vi "DefendAreaTactic.vi"(6 "Number of Defenders\nWithout Duelist":i32, 7 "First call?":bool, 8 "error in (no error)":errorcluster, 9 "Robot":refnum<class "Robot.lvclass">, 10 "Game in":refnum<class "Game.lvclass">, 11 "DefendAreaTactic in":refnum<class "DefendAreaTactic.lvclass">) -> (0 "error out":errorcluster, 2 "Robot out":refnum<class "Robot.lvclass">, 3 "DefendAreaTactic out":refnum<class "DefendAreaTactic.lvclass">)   [LabVIEW 2024, in "DefendAreaTactic.lvclass"]
uses:
  DefendAreaTactic.lvclass
  C:/Users/moise/Documents/GitHub/SSL_AI/Tactic_class/Tactic.lvclass
  Robot_class/Robot.lvclass
  C:/Users/moise/Documents/GitHub/SSL_AI/Object_class/Object.lvclass
  Game_class/Game.lvclass
  Robot_class/tactics.ctl
  DefendAreaTacticStates.ctl
  Robot_class/robotKickToStates.ctl
  Tactic_class/Tactic.lvclass/Tactic.ctl
  WallPositions.ctl
  Robot_class/Robot.lvclass/Robot.ctl
  Object_class/Object.lvclass/Object.ctl
  Game_class/Game.lvclass/Game.ctl
  Team_class/Team.lvclass/Team.ctl
  Ball_class/Ball.lvclass/Ball.ctl
  Field_class/Field.lvclass/Field.ctl
  Parameters_class/Parameters.lvclass/Parameters.ctl
  Skillbook_class/Skillbook.lvclass/Skillbook.ctl
  DefendAreaTactic.lvclass/DefendAreaTactic.ctl
  <vilib>/Analysis/_algsub.llb/Real Vector Norm.vi
  Game_class/Read DefensiveTeam.vi
  Game_class/Read BallRef.vi
  Game_class/Read FieldRef.vi
  Game_class/Read NewParameters.vi
  Field_class/Read ourGoalPosition.vi
  Ball_class/Read v_x.vi
  Ball_class/Read v_y.vi
  Object_class/Read x.vi
  Object_class/Read y.vi
  Object_class/Read position(x,y).vi
  Ball_class/Read velocityNorm.vi
  Team_class/Read RobotRef.vi
  Robot_class/Read id.vi
  Robot_class/Write dest_x.vi
  Robot_class/Write dest_y.vi
  Robot_class/Write dest_orientation.vi
  Game_class/Read OffensiveTeam.vi
  Game_class/Read EnemyRef.vi
  Game_class/Read Parameters.lvclass.vi
  Game_class/Read Utilities.lvclass.vi
  Parameters_class/Read AttakingOurselves.vi
  Skillbook_class/Read HaltSkill.vi
  Tactic_class/Read Skillbook.vi
  Write States.vi
  Robot_class/Write tactic.vi
  Robot_class/Write keepDest.vi
  Robot_class/Write robotKickState.vi
  Ball_class/Ball.lvclass
  Ally_class/Ally.lvclass
  C:/Users/moise/Documents/GitHub/SSL_AI/Team_class/Team.lvclass
  Enemy_class/Enemy.lvclass
  Skillbook_class/Skillbook.lvclass
  Field_class/Field.lvclass
  Parameters_class/Parameters.lvclass
  Utilities_class/Utilities.lvclass
  HaltSkill_class/HaltSkill.lvclass
  DefendGoalTactic_class/DefendGoalTactic.lvclass
  <vilib>/Analysis/NI_AALPro.lvlib
  <vilib>/Analysis/coordinate.llb/2D Cartesian Coordinate Rotation (Scalar).vi
  Team_class/Team.lvclass
  <vilib>/Analysis/NI_AALBLAS.lvlib
panel:
  out "x .or. y?":bool
  out "Dist":dbl
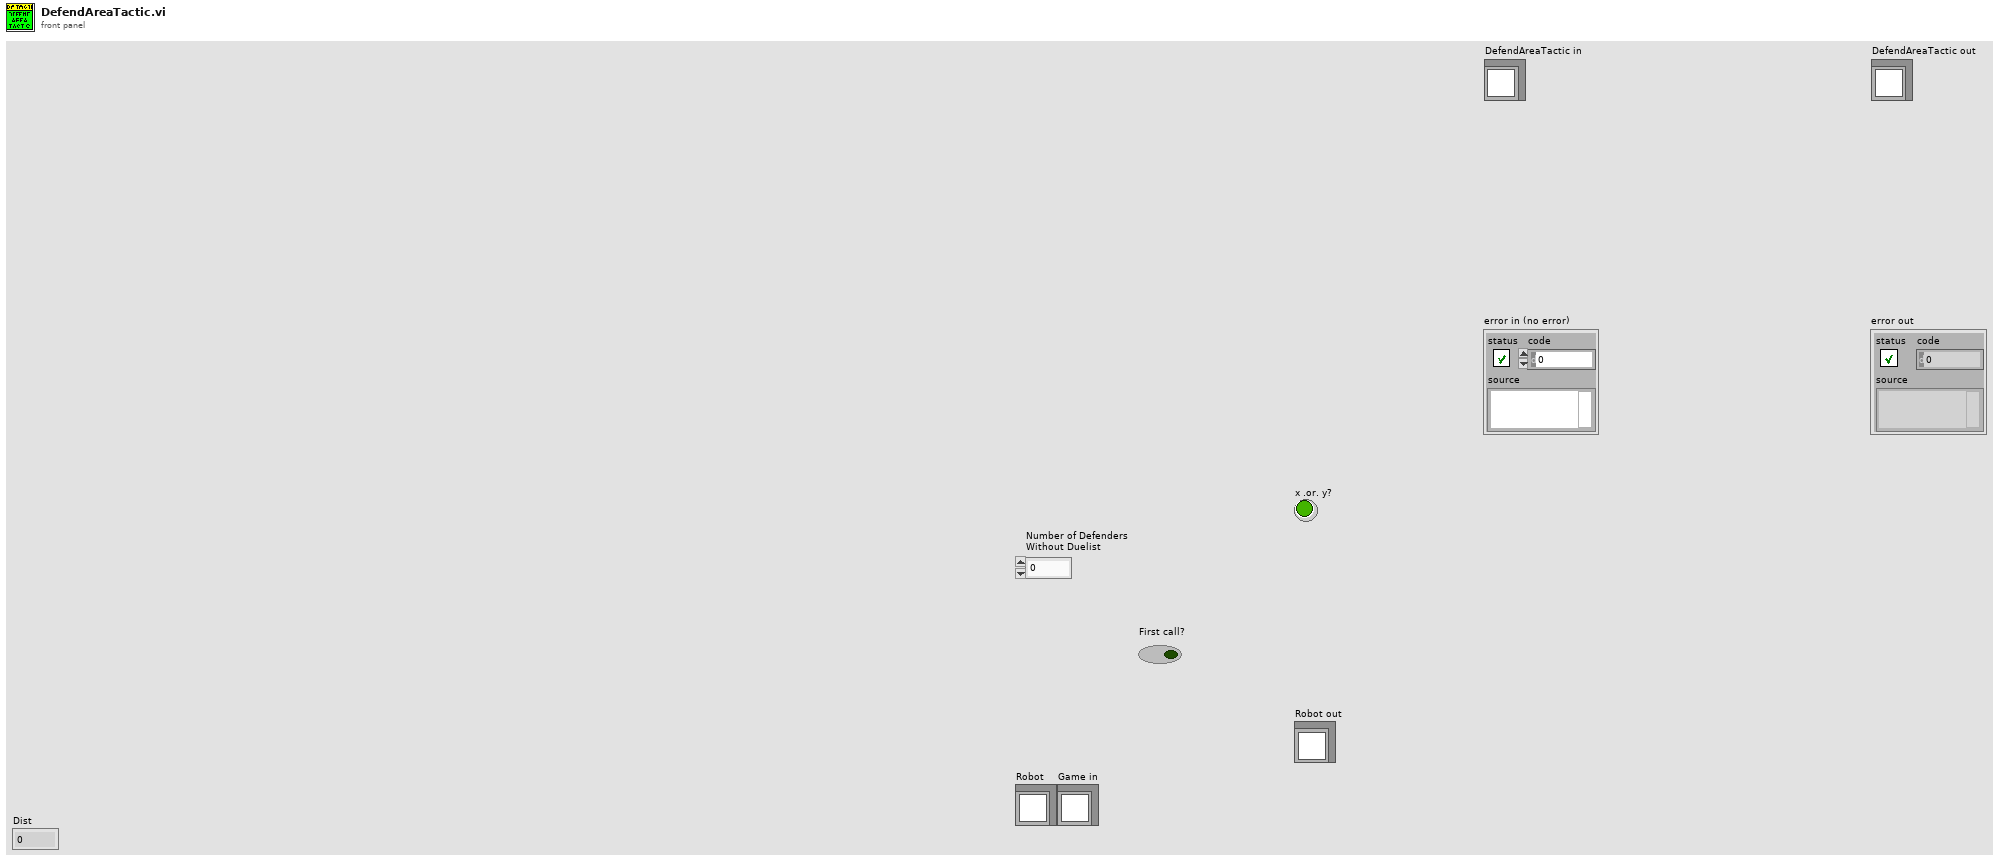
[diagram p1: front panel]
types:
  T1 = typedef "robotKickToStates.ctl" = enum16{"shootFromDirect", "avoidCollideBall", "goToBackBall", "none", "walk", "turn", "turnAntiClockWise", "turnClockwise", "oldKickToShoot", "oldKickToGoToBackBall", "shoot"}
  T2 = typedef "DefendAreaTactic.lvclass/DefendAreaTacticStates.ctl" = enum16{"BlockShot", "BlockPossibleShot", "CoverOneTouchShot", "BallInKeeperArea", "Exit"}
  T3 = typedef "tactics.ctl" = enum16{"GoToBallPlacementPosition", "PlaceBall", "GoToBallPlacement", "5Robots", "BallPlacementEnemy", "ReceivePassInFuturePoint", "Roller", "PrepareRollToPassRollerGoTo", "PrepareRollToPassReceiverGoTo", "WaitRoll", "PositionToRoll", "PenaltyAttacker", "PassObserver", "PenaltyDefense", "TableReceiverTactic", "Test", "DefendGoal", "Marker", "FollowAttacker", "DefendArea", "Shoot", "AttackerAimGoal", "AttackerBallOutOfField", "AttackerBlock", "AttackerStop", "Duelist", "Halt", "ZigZag", "GoTo", "Timeout", "KickToBestRobot", "KickToPassReceiver", "PositionToReceivePass", "WaitPass", "GoToTarget"}
  T4 = typedef "WallPositions.ctl" = enum16{"LeftWall", "LeftCorner", "FrontWall", "RightCorner", "RightWall"}
  T5 = typedef "NewParameters.ctl" = cluster{"PenaltyDistance":dbl, "DistanceAttackerToBackBall":dbl, "Division":enum16{"Div B", "Div A"}, "DistanceToAvoidyEnemyRobot":dbl, "BallPlacementDistance":dbl, "DisatanceBehindBallToStealBall":dbl, "MaxDistanceToPositionKickoff":dbl, "BlockEnemyTarget":bool, "MaxStopVAng":dbl, "DistanceMarkerToEnemy":dbl, "IgnoreDribblerContact":bool, "DistanceToBeginEnemyPosession":dbl, "GoToBallWhenEnemyNotMoving":bool, "EnemyDistanceToReduceVelocity":dbl, "TurnOnEnemyDistanceToReduceVelocity":bool, "EnemyDistanceToShootOutBall":dbl, "DefenseKickBall":bool, "MoreKickToGoal? (0-0.3)":dbl, "ChipKickInEnemyField":bool, "ShootOutRobotId":dbl, "FieldLenghtDenominatorInShootOut":dbl, "AdjustPositionInBallPlacement":bool, "PowerGodPass":dbl, "VelocityAbortEnemyPos":dbl, "MaxDistToBeginPass":dbl, "MinDistToBeginPass":dbl, "VelocityInDirects":dbl, "BadDribblerIDs":i32[], "NewKickToDistanceAroundBall":dbl, "PowerAvoidColisionMarker":dbl, "DistanceToAvoidColisionMarker":dbl, "AvoidBallKick":dbl, "DistanceTryKick":dbl, "SuicideKickDIstance":dbl, "AdjustFirstKickDistance":dbl, "AvoidAimLessKick":dbl, "DistanceToAvoidyEnemyShootRobot ":dbl, "NumberOfMarkers":dbl, "PotField":bool, "PIDLateral":bool, "MinDistanceFirstKickX":dbl, "MinDistanceFirstKickY":dbl, "FractionOfDistToTouchGround\nAfterChipKick":dbl, "FractionOfKickxWhen\nComposedWithKickz":dbl, "Style":T6, "MoveInTurnState":bool, "DistFromEnemyToConsider\nMoveInTurnState":dbl, "CascadePID":bool, "TurnAroundParameters":cluster{"Radius":dbl, "Multiplier":dbl, "ChordAngle":dbl}, "SafeDriveVel":dbl, "DistanceToGoToBackBall":dbl, "minDistanceToNotFinish\nEnemyPossession":dbl, "OneTouchShot":cluster{"angleFactor":dbl, "maxAngle":dbl, "Attack":bool, "Defense":bool}, "OpenAngleToGoal":cluster{"minAngle":dbl, "maxAngle":dbl, "minEvaluation":dbl}, "ShotInterception":cluster{"shotSpeed":dbl, "minEnemySpeed":dbl, "maxEnemySpeed":dbl, "minEvaluation":dbl}, "AllyTeamArray":T7[], "maxDefendersNumber":i32, "Zone":cluster{"GuardPositionArray":dbl[][], "ZoneMidField":dbl[], "CenterForwardWidth":dbl}, "MinEvaluationToShoot":dbl, "PassInterception":cluster{"maxPassSpeed":dbl, "minPassSpeed":dbl, "minEnemySpeed":dbl, "chipPassDistance":dbl, "chipPassEvaluation":dbl, "minEvaluation":dbl, "maxEnemySpeed":dbl}, "PassDistance":cluster{"maxDistance":dbl, "minDistance":dbl}, "receiverSpeed":dbl, "maxBallSpeed":dbl, "slackTime":dbl, "Turning radius":dbl, "Turning v_ang":dbl, "AlignError":cluster{"Distance":dbl, "Orientation":dbl, "V_norm(m/s)":dbl, "V_ang (rad/s)":dbl}, "RobotRadius":dbl, "KickerDistance":dbl, "keeper angle  to cover goalpost":dbl, "a_slide":dbl, "a_roll":dbl, "k_switch":dbl}
  T6 = typedef "Style.ctl" = enum16{"Insanity", "Offensive", "Defensive"}
  T7 = typedef "AllyTeam.ctl" = enum16{"Keeper", "Defender", "Attacker"}
  T8 = typedef "DefendGoalTactic.lvclass/DefendGoalTacticStates.ctl" = enum16{"BlockShot", "BlockPossibleShot", "CoverOneTouchShot", "Kick", "GuardGoal", "Exit"}
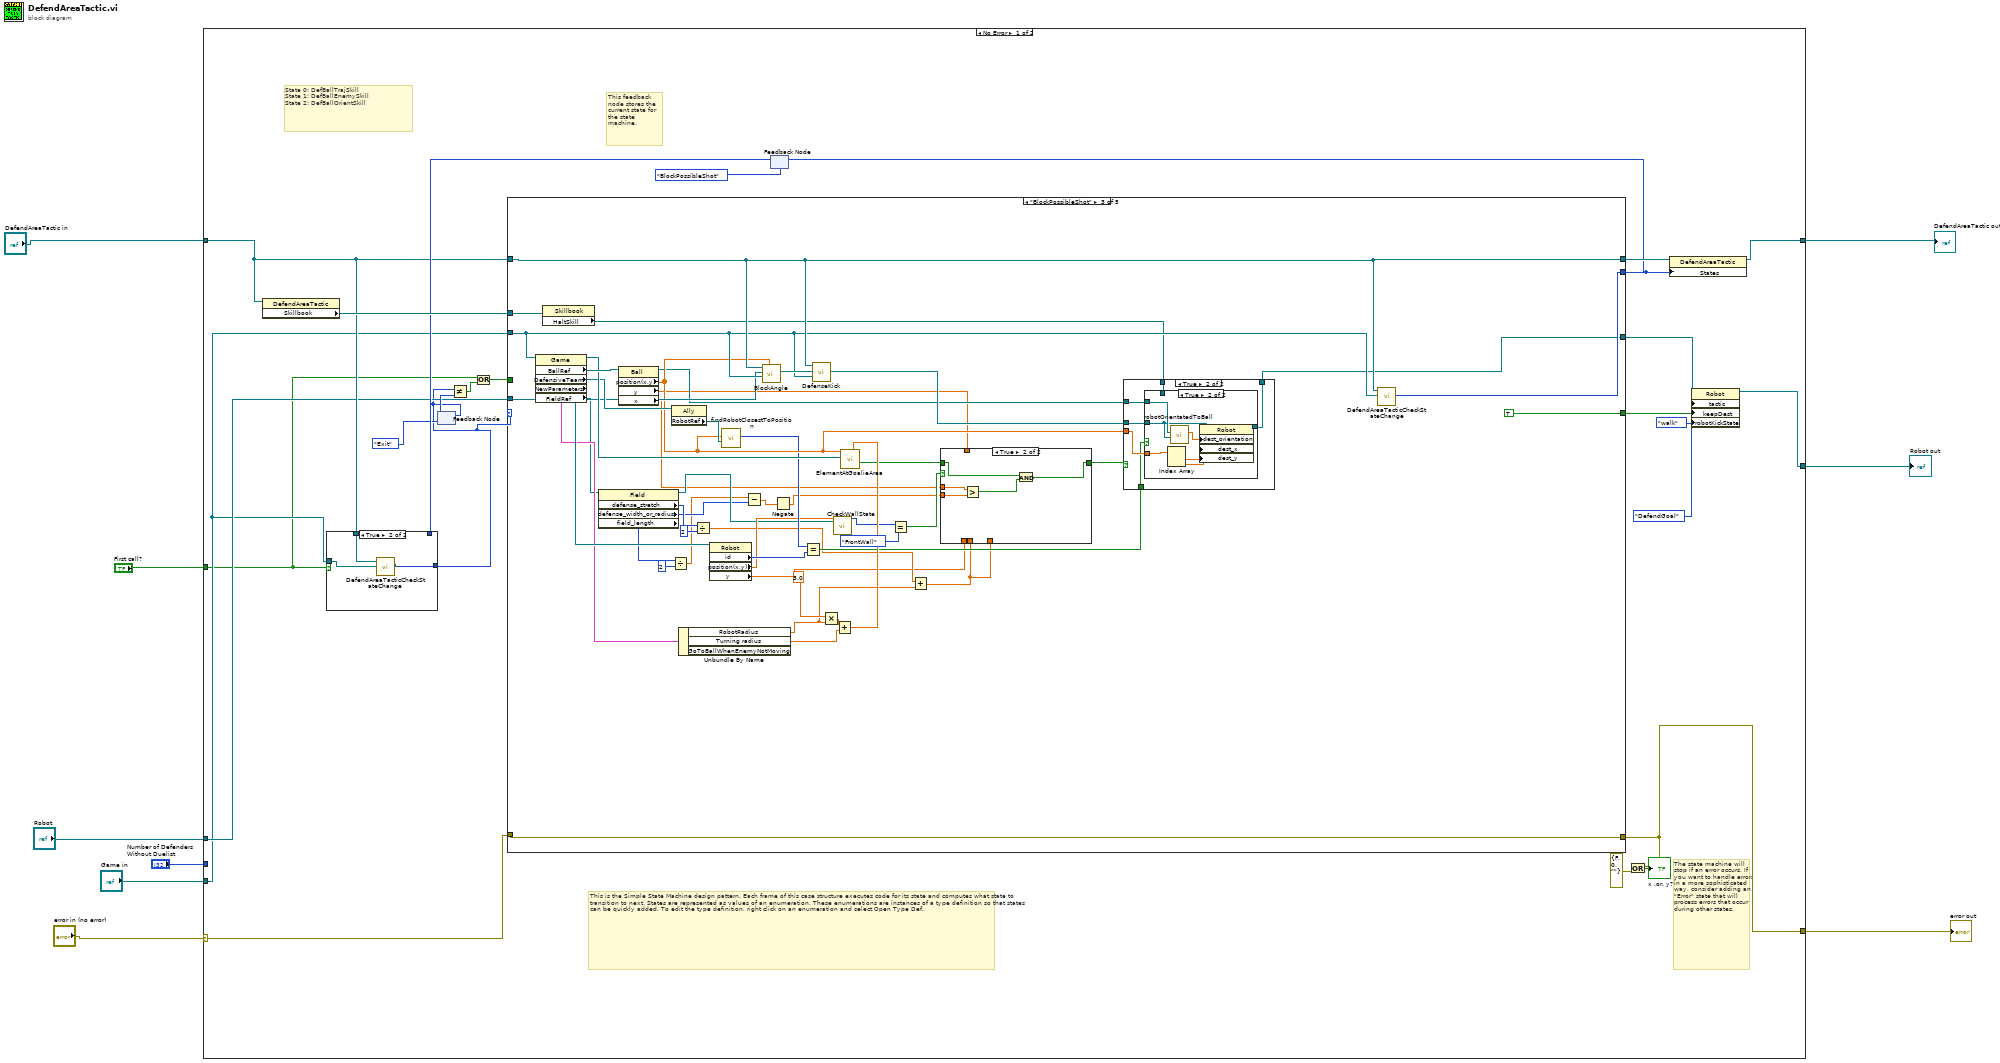
[diagram p0: block diagram]
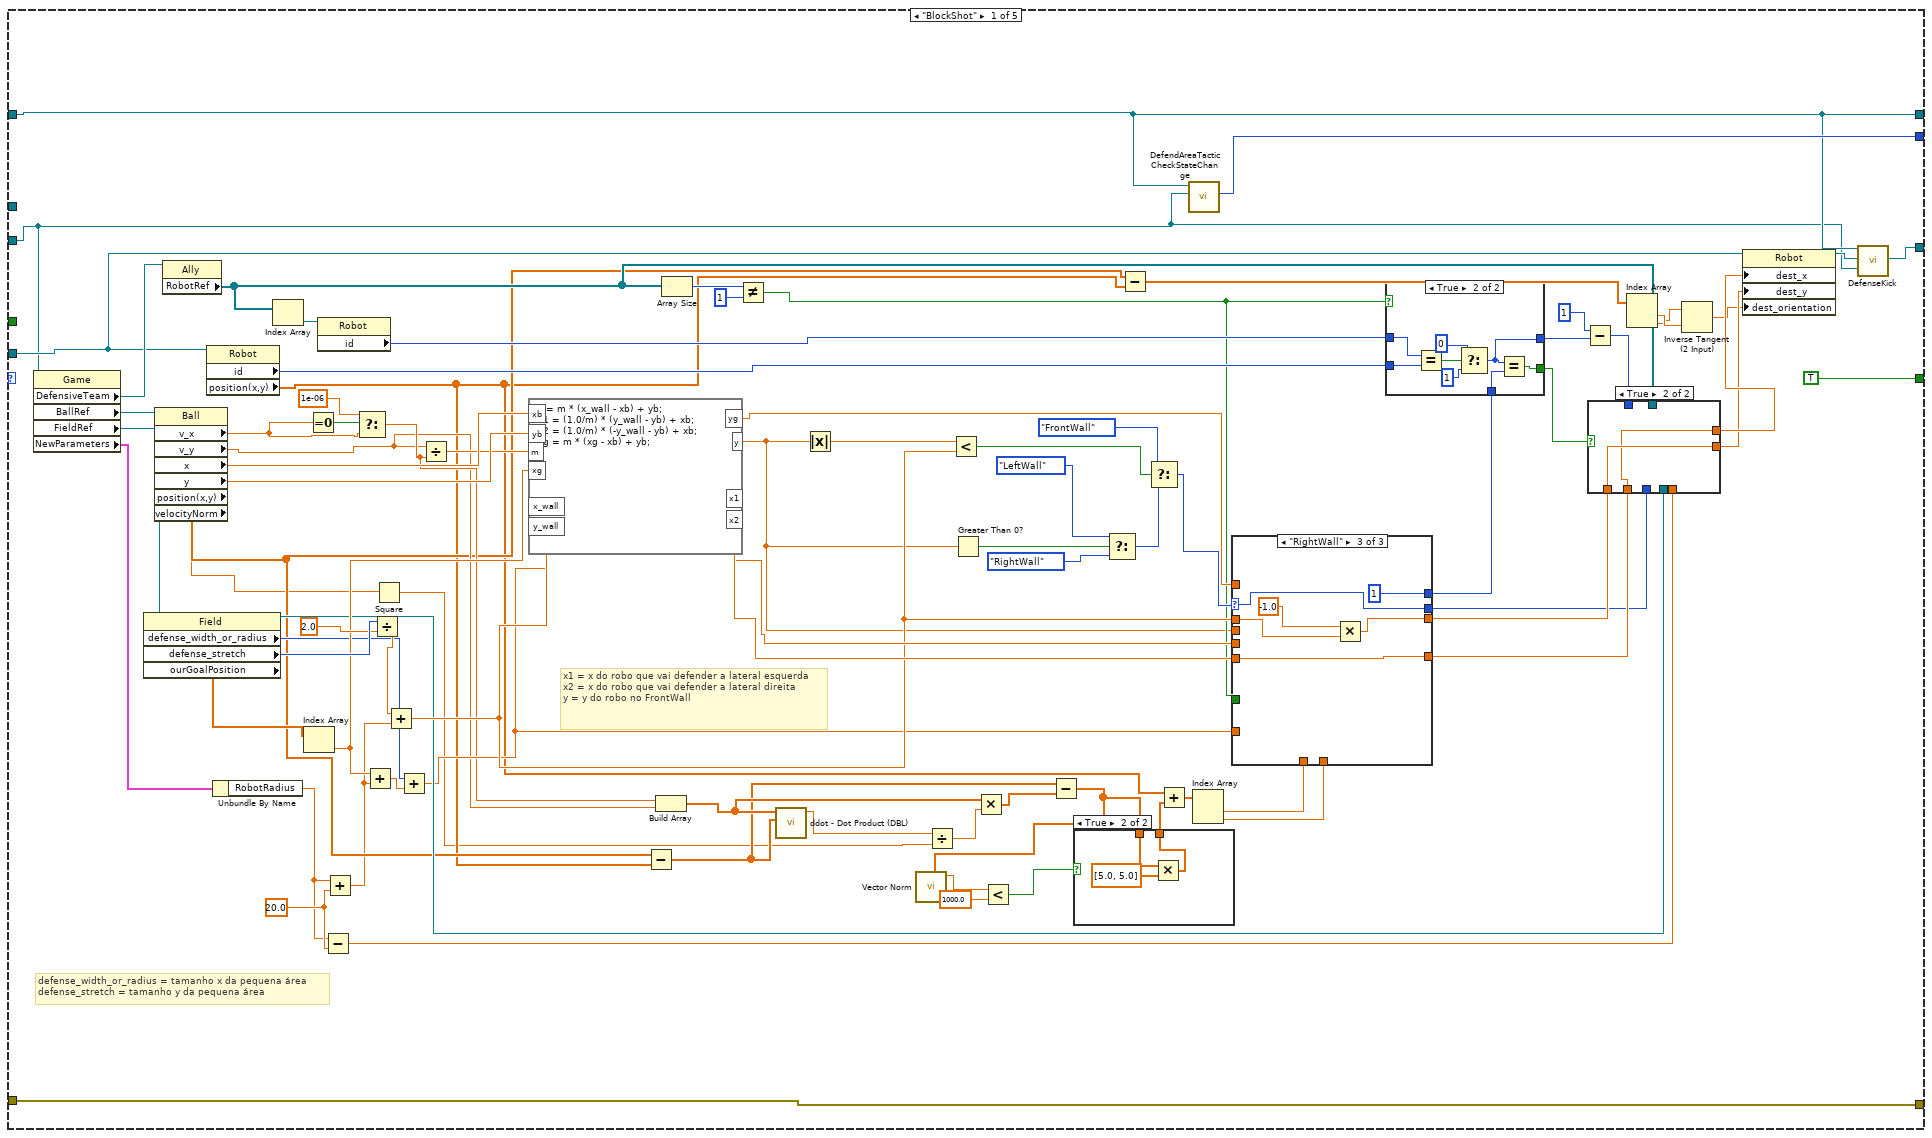
[diagram p3: hidden frame]
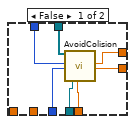
[diagram p5: hidden frame]
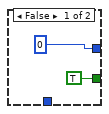
[diagram p6: hidden frame]
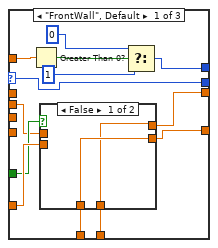
[diagram p7: hidden frame]
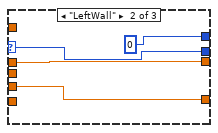
[diagram p9: hidden frame]
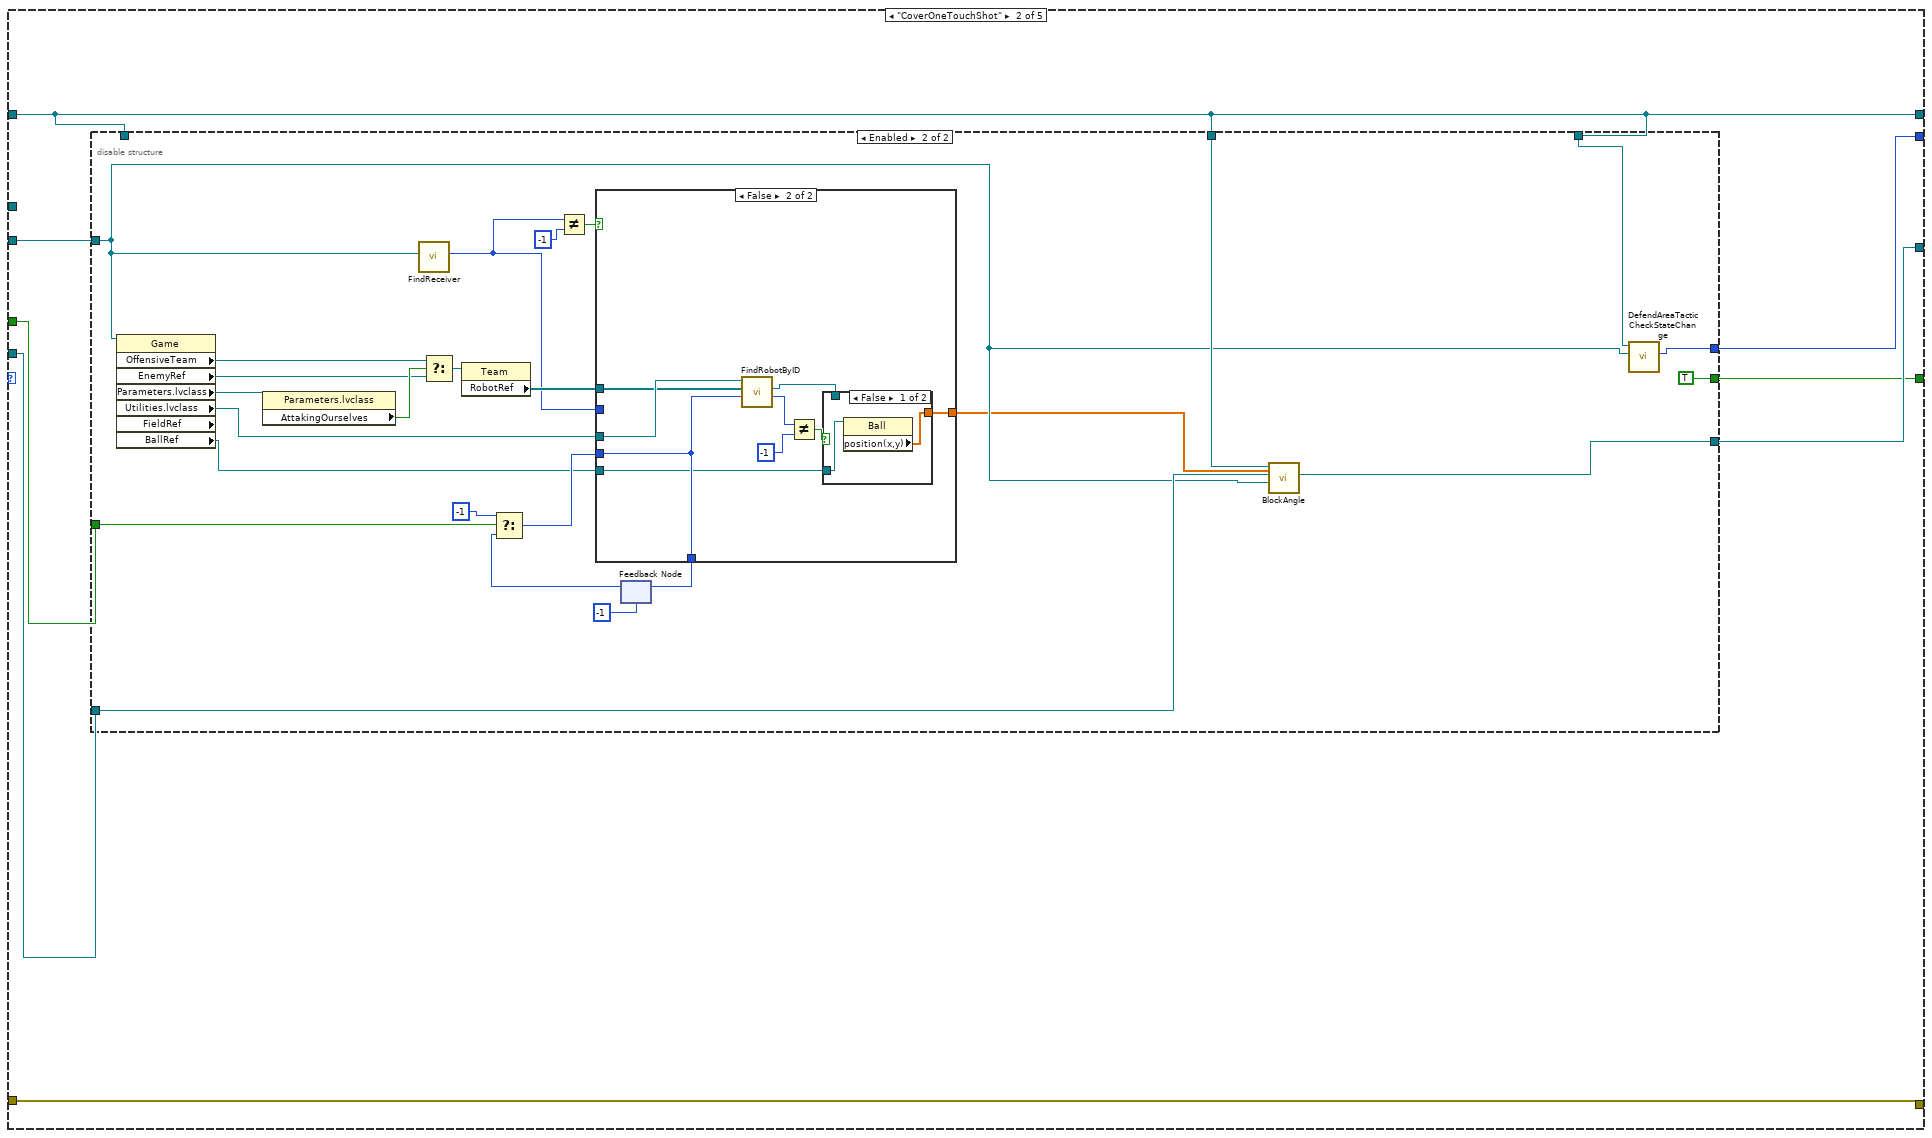
[diagram p10: hidden frame]
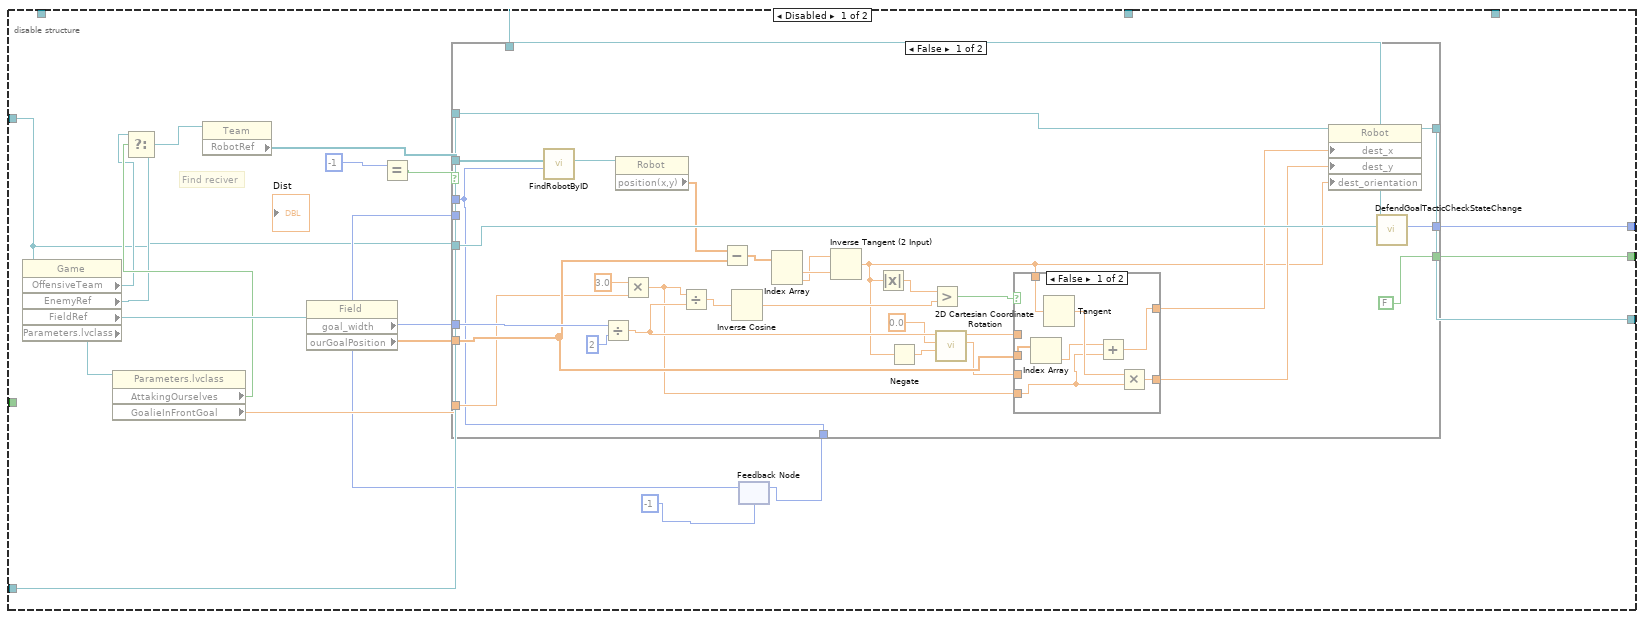
[diagram p11: hidden frame]
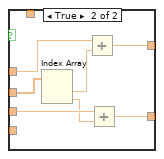
[diagram p12: hidden frame]
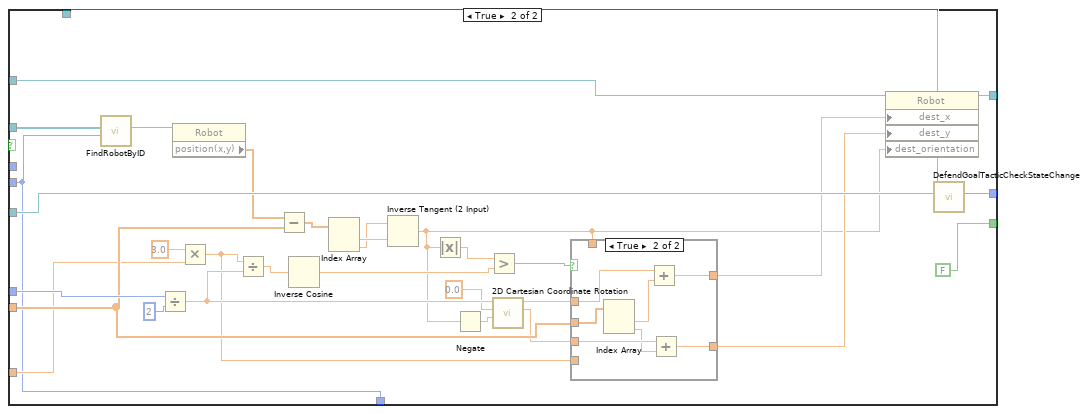
[diagram p13: hidden frame]
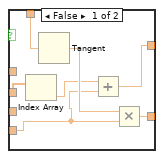
[diagram p14: hidden frame]
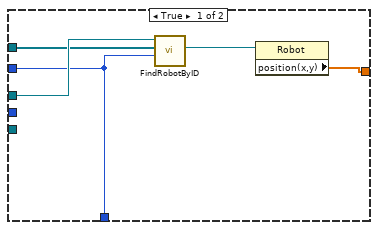
[diagram p15: hidden frame]
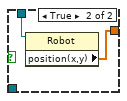
[diagram p16: hidden frame]
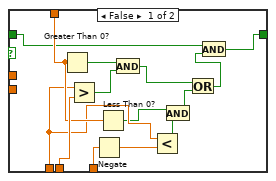
[diagram p17: hidden frame]
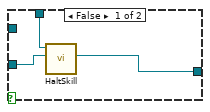
[diagram p19: hidden frame]
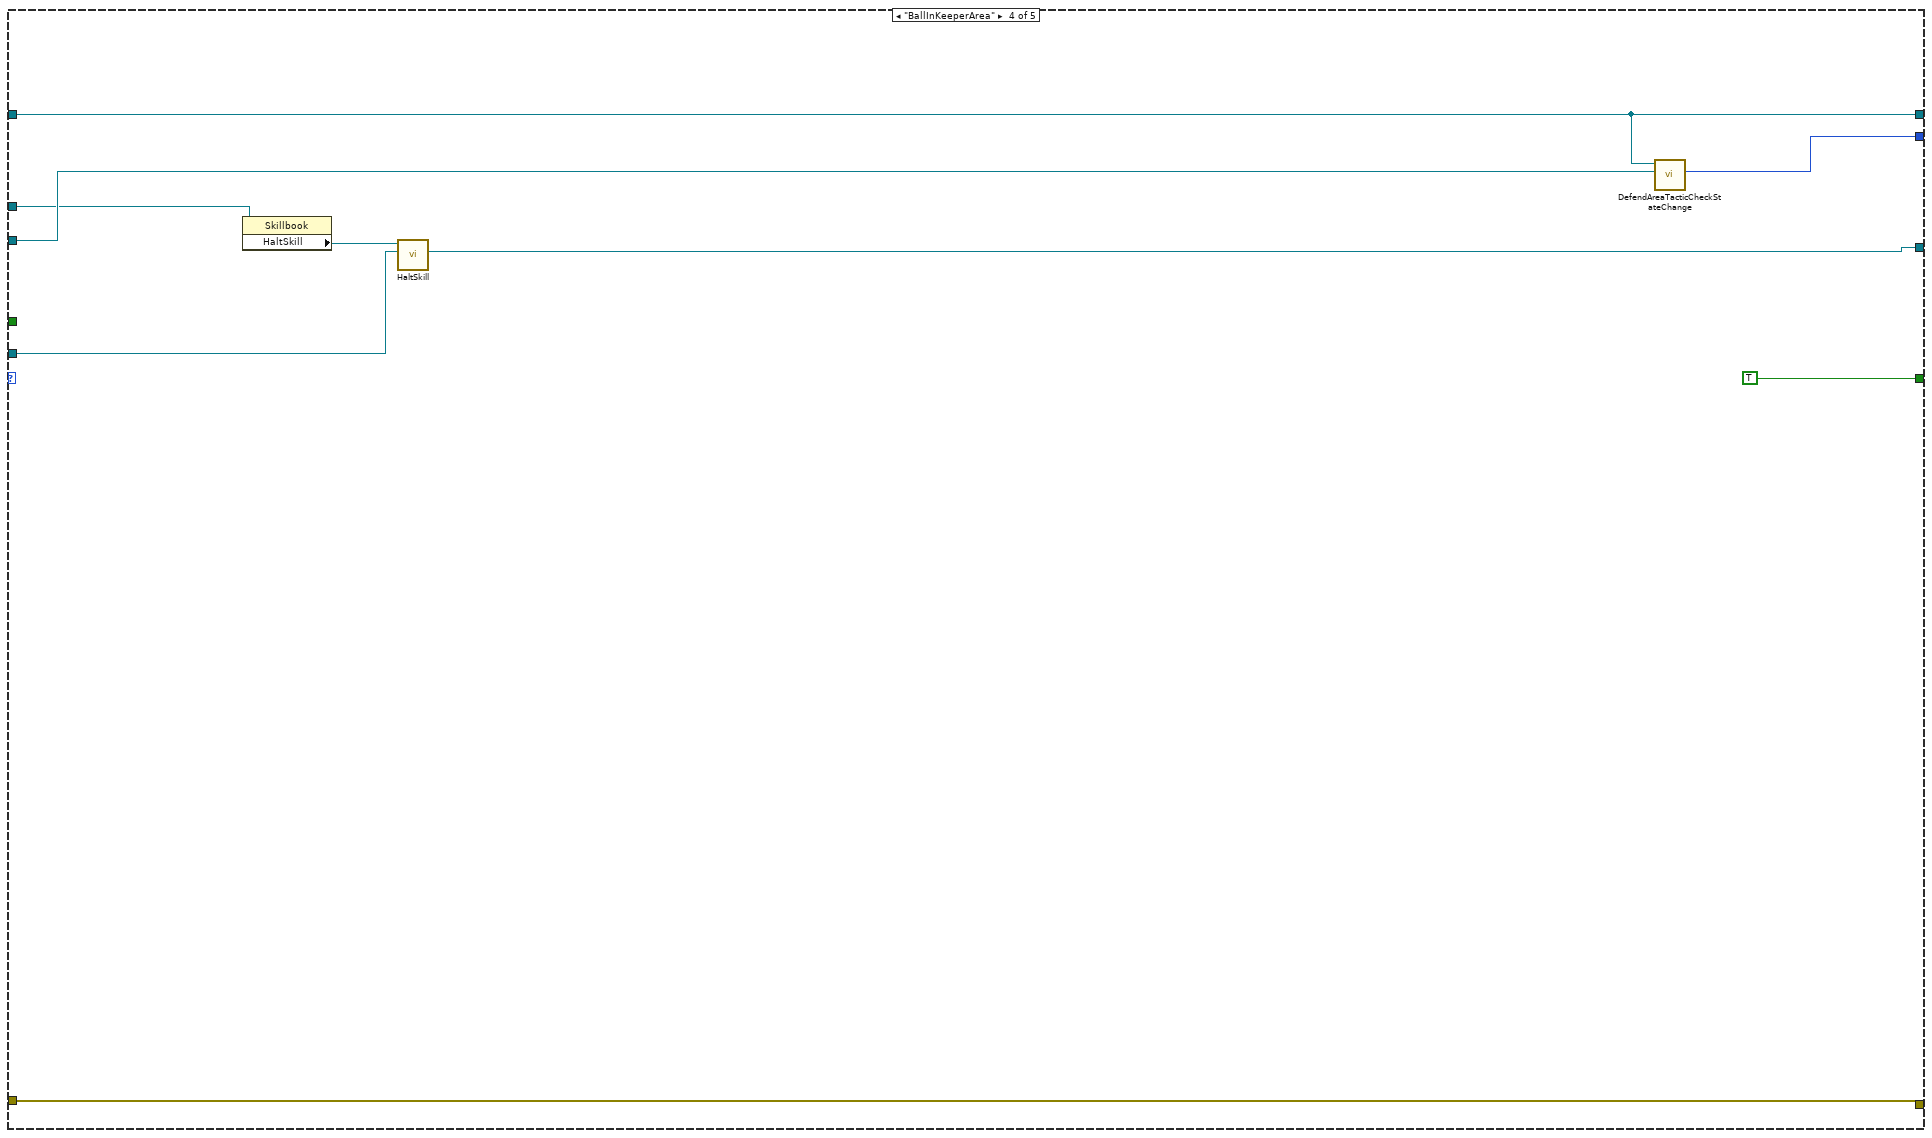
[diagram p20: hidden frame]
diagram:
  n1 = case shown="No Error" "error in (no error)" {
    selector: "error in (no error)" -> [w19 w433]
    tunnel: [w15 w433] -> w4
    tunnel: [w21 w432] -> w3
    tunnel: "DefendAreaTactic in" -> [w22 w432]
    tunnel: "Robot" -> [w18 w431]
    tunnel: [w20 w431] -> w8
    tunnel: "Game in" -> [w17 _]
    tunnel: "Number of Defenders\nWithout Duelist" -> [_ _]
    tunnel: "First call?" -> [w16 _]
    frame No Error {
      # "State 0: DefBallTrajSkill\nState 1: DefBallEnemySkill\nState 2: DefBallOrientSkill"
      # "The state machine will stop if an error occurs. If you want to handle errors in a more sophisticated way, consider adding an \"Error\" state that will process errors that occur during other states."
      # "This feedback node stores the current state for the state machine."
      # "This is the Simple State Machine design pattern. Each frame of this case structure executes code for its state and computes what state to transition to next. States are represented as values of an enumeration. These enumerations are instances of a type definition so that states can be quickly added. To edit the type definition, right click on an enumeration and select Open Type Def."
      n2 = property class="DefendAreaTactic"(reference=w22) -> ("Skillbook"=w32:refnum<class "Skillbook.lvclass">)  [unwired: 1 in, 2 out]
      n3 = feedback #1(DefendAreaTacticStates."Exit" ("States")) -> (w24:T2)
      n4 = feedback #2(DefendAreaTacticStates."BlockPossibleShot" ("States")) -> (w30:T2)
      n5 = case shown="True" w16 {
        tunnel: [w34 w35] -> w11
        tunnel: w30 -> [w34 _]
        tunnel: w17 -> [_ w37]
        tunnel: w22 -> [_ w36]
        frame False {
        }
        frame True {
          n6 = call "DefendAreaTacticCheckStateChange.vi"("Game"=w37, "DefendAreaTactic in"=w36) -> ("States"=w35:T2)  [unwired: 7 in, 2 out]
        }
      }
      n7 = feedback-in #1(w11) -> ()
      n8 = Not Equal?(x=w11, y=w24) -> (x != y?=w25:bool)
      n9 = Or(x=w16, y=w25) -> (x .or. y?=w26:bool)
      n10 = case shown="\"BlockPossibleShot\"" w11 {
        tunnel: w19 -> [w121 w179 w380 w425 w430]
        tunnel: [w121 w179 w380 w425 w430] -> w15
        tunnel: w32 -> [_ _ w357 w420 _]
        tunnel: w18 -> [w88 w176 w371 w418 w426]
        tunnel: [w74 w177 w368 w417 w426] -> w27
        tunnel: [w77 w172 w377 w422 w427] -> w31
        tunnel: w22 -> [w77 w172 w377 w422 w427]
        tunnel: w17 -> [w75 w178 w375 w421 _]
        tunnel: [w119 w174 w379 w423 DefendAreaTacticStates."Exit" ("States")] -> w14
        tunnel: w26 -> [_ w173 _ _ _]
        tunnel: [TRUE ("keepDest") w175 TRUE TRUE ("keepDest") TRUE ("keepDest")] -> w23
        frame "BlockShot" {
          w83 = 20.0
          # "x1 = x do robo que vai defender a lateral esquerda\nx2 = x do robo que vai defender a lateral direita\ny = y do robo no FrontWall"
          # "defense_width_or_radius = tamanho x da pequena área\ndefense_stretch = tamanho y da pequena área"
          n11 = property class="Game"(reference=w75) -> ("DefensiveTeam"=w95:refnum<class "Ally.lvclass">, "BallRef"=w118:refnum<class "Ball.lvclass">, "FieldRef"=w115:refnum<class "Field.lvclass">, "NewParameters"=w114:T5)  [unwired: 1 in, 2 out]
          n12 = property class="Field"(reference=w115) -> (reference out=w81:refnum<class "Field.lvclass">, "defense_width_or_radius"=w72:i32, "defense_stretch"=w113:i32, "ourGoalPosition"=w111:dbl[])  [unwired: 1 in, 1 out]
          n13 = property class="Ball"(reference=w118) -> ("v_x"=w69:dbl, "v_y"=w57:dbl, "x"=w117:dbl, "y"=w116:dbl, "position(x,y)"=w56:dbl[], "velocityNorm"=w46:dbl)  [unwired: 1 in, 2 out]
          n14 = property class="Ally"(reference=w95) -> ("RobotRef"=w80:refnum<class "Robot.lvclass">[])  [unwired: 1 in, 2 out]
          n15 = property class="Robot"(reference=w88) -> ("id"=w92:i32, "position(x,y)"=w50:dbl[])  [unwired: 1 in, 2 out]
          n16 = Unbundle By Name(w114) -> ("RobotRadius"=w39:dbl)
          n17 = Index Array(array=w80) -> (element=w94:refnum<class "Robot.lvclass">)  [unwired: 1 in]
          n18 = Index Array(array=w111) -> (element=w98:dbl)  [unwired: 1 in]
          n19 = Equal To 0?(x=w69) -> (x = 0?=w71:bool)
          n20 = property class="Robot"(reference=w94) -> ("id"=w93:i32)  [unwired: 1 in, 2 out]
          n21 = Subtract(x=w39, y=w83) -> (x-y=w82:dbl)
          n22 = Add(x=w39, y=w83) -> (x+y=w40:dbl)
          n23 = Select(t=1e-06, s=w71, f=w69) -> (s? t:f=w58:dbl)
          n24 = Add(x=w98, y=w40) -> (x+y=w73:dbl)
          n25 = Divide(x=w113, y=2.0) -> (x/y=w110:dbl)
          n26 = Square(x=w46) -> (x^2=w45:dbl)
          n27 = Add(x=w110, y=w40) -> (x+y=w99:dbl)
          n28 = Add(x=w72, y=w73) -> (x+y=w60:dbl)
          n29 = Divide(x=w57, y=w58) -> (x/y=w65:dbl)
          n30 = formula code="y = m * (x_wall - xb) + yb;\nx1 = (1.0/m) * (y_wall - yb) + xb;\nx2 = (1.0/m) * (-y_wall - yb) + xb;\nyg = m * (xg - xb) + yb;"("xb"=w117, "yb"=w116, "x_wall"=w60, "y_wall"=w99, "m"=w65, "xg"=w98) -> ("y"=w59:dbl, "x1"=w100:dbl, "x2"=w101:dbl, "yg"=w68:dbl)
          n31 = Subtract(x=w56, y=w50) -> (x-y=w51:dbl[])
          n32 = Build Array(w58, w57) -> (w54:dbl[])
          n33 = Array Size(array=w80) -> (size(s)=w97:i32)
          n34 = Not Equal?(x=w97, y=1) -> (x != y?=w66:bool)
          n35 = call <vilib>:"ddot - Dot Product (DBL).vi"("y"=w51, "x"=w54) -> ("ddot"=w55:dbl)  [unwired: 8 in, 1 out]
          n36 = Absolute Value(x=w59) -> (abs(x)=w109:dbl)
          n37 = Divide(x=w55, y=w45) -> (x/y=w53:dbl)
          n38 = Less?(x=w109, y=w99) -> (x < y?=w108:bool)
          n39 = Greater Than 0?(x=w59) -> (x > 0?=w103:bool)
          n40 = Multiply(x=w54, y=w53) -> (x*y=w52:dbl[])
          n41 = Subtract(x=w51, y=w52) -> (x-y=w42:dbl[])
          n42 = call-poly <vilib>:"Vector Norm.vi"("Input Vector"=w42) -> ("norm"=w44:dbl)  [unwired: 9 in, 1 out]
          n43 = Less?(x=w44, y=1000.0) -> (x < y?=w43:bool)
          n44 = case shown="True" w43 {
            tunnel: w42 -> [w122 w125]
            tunnel: [w122 w124] -> w41
            frame False {
            }
            frame True {
              n45 = Multiply(x=w125, y=dbl[] [5.0, 5.0]) -> (x*y=w124:dbl[])
            }
          }
          n46 = Select(t=WallPositions."LeftWall", s=w103, f=WallPositions."RightWall") -> (s? t:f=w105:T4)
          n47 = Subtract(x=w56, y=w50) -> (x-y=w61:dbl[])
          n48 = Select(t=WallPositions."FrontWall", s=w108, f=w105) -> (s? t:f=w104:T4)
          n49 = Add(x=w50, y=w41) -> (x+y=w49:dbl[])
          n50 = call "DefendAreaTacticCheckStateChange.vi"("Game"=w75, "DefendAreaTactic in"=w77) -> ("States"=w119:T2)  [unwired: 7 in, 2 out]
          n51 = Index Array(array=w49) -> (element #1=w48:dbl, element #2=w47:dbl)  [unwired: 2 in]
          n52 = case shown="\"RightWall\"" w104 {
            selector: w104 -> [w152 w162 w166]
            tunnel: w59 -> [w148 _ _]
            tunnel: w100 -> [_ w164 _]
            tunnel: w101 -> [_ _ w168]
            tunnel: w99 -> [_ w165 w170]
            tunnel: w60 -> [w151 _ _]
            tunnel: [w147 w165 w169] -> w86
            tunnel: [w150 w164 w168] -> w85
            tunnel: [w153 0 1] -> w89
            tunnel: w68 -> [w157 _ _]
            tunnel: [w152 w162 w166] -> w78
            tunnel: w66 -> [w149 _ _]
            tunnel: w48 -> [w146 _ _]
            tunnel: w47 -> [w145 _ _]
            frame "FrontWall", Default {
              n53 = Greater Than 0?(x=w157) -> (x > 0?=w156:bool)
              n54 = case shown="False" w149 {
                tunnel: w151 -> [_ w161]
                tunnel: [w159 w161] -> w150
                tunnel: w148 -> [_ w160]
                tunnel: [w158 w160] -> w147
                tunnel: w146 -> [w159 _]
                tunnel: w145 -> [w158 _]
                frame False {
                }
                frame True {
                }
              }
              n55 = Select(t=0, s=w156, f=1) -> (s? t:f=w153:i32)
            }
            frame "LeftWall" {
            }
            frame "RightWall" {
              n56 = Multiply(x=-1.0, y=w170) -> (x*y=w169:dbl)
            }
          }
          n57 = case shown="True" w66 {
            tunnel: w93 -> [_ w141]
            tunnel: w92 -> [_ w140]
            tunnel: w89 -> [_ w139]
            tunnel: [TRUE w138] -> w87
            tunnel: [0 ("Numeric") w137] -> w91
            frame False {
            }
            frame True {
              n58 = Equal?(x=w141, y=w140) -> (x = y?=w144:bool)
              n59 = Select(t=0, s=w144, f=1) -> (s? t:f=w137:i32)
              n60 = Equal?(x=w137, y=w139) -> (x = y?=w138:bool)
            }
          }
          n61 = Subtract(x=1, y=w91) -> (x-y=w79:i32)
          n62 = case shown="True" w87 {
            tunnel: w86 -> [_ w134]
            tunnel: w85 -> [_ w133]
            tunnel: [w129 w133] -> w84
            tunnel: [w128 w134] -> w67
            tunnel: w82 -> [w132 _]
            tunnel: w81 -> [w131 _]
            tunnel: w80 -> [w130 _]
            tunnel: w79 -> [w127 _]
            tunnel: w78 -> [w126 _]
            frame False {
              n63 = call "AvoidColision.vi"("RobotRef"=w130, "referencia"=w127, "positionOnWall"=w126, "Field"=w131, "robot Radius"=w132) -> ("dest_x"=w129:dbl, "dest_y"=w128:dbl)  [unwired: 12 in, 1 out]
            }
            frame True {
            }
          }
          n64 = Index Array(array=w61) -> (element #1=w64:dbl, element #2=w63:dbl)  [unwired: 2 in]
          n65 = Inverse Tangent (2 Input)(1:w64, 2:w63) -> (0:w62:dbl)
          n66 = property class="Robot"(reference=w88, "dest_x"=w84, "dest_y"=w67, "dest_orientation"=w62) -> (reference out=w76:refnum<class "Robot.lvclass">)  [unwired: 1 in, 1 out]
          n67 = call "DefenseKick.vi"("object in"=w77, "Robot"=w76, "Game"=w75) -> ("Robot out"=w74:refnum<class "Robot.lvclass">)  [unwired: 14 in, 2 out]
        }
        frame "CoverOneTouchShot" {
          n68 = disable-structure shown="Enabled" {
            disable-tunnel: w172 -> [w200 _]
            disable-tunnel: w178 -> [w180 w293]
            disable-tunnel: [w198 w292] -> w177
            disable-tunnel: w176 -> [w197 w294]
            disable-tunnel: [w192 w296] -> w174
            disable-tunnel: [w188 TRUE ("keepDest")] -> w175
            disable-tunnel: w172 -> [_ w297]
            disable-tunnel: w173 -> [_ w303]
            disable-tunnel: w172 -> [_ w295]
            frame Disabled {
              # "Find reciver"
              n69 = property class="Game"(reference=w180) -> ("OffensiveTeam"=w181:refnum<class "Ally.lvclass">, "EnemyRef"=w182:refnum<class "Enemy.lvclass">, "FieldRef"=w196:refnum<class "Field.lvclass">, "Parameters.lvclass"=w190:refnum<class "Parameters.lvclass">)  [unwired: 1 in, 2 out]
              n70 = property class="Parameters.lvclass"(reference=w190) -> ("AttakingOurselves"=w184:bool, "GoalieInFrontGoal"=w189:dbl)  [unwired: 1 in, 2 out]
              n71 = Select(t=w181, s=w184, f=w182) -> (s? t:f=w183:refnum<class "Team.lvclass">)
              n72 = property class="Team"(reference=w183) -> ("RobotRef"=w199:refnum<class "Robot.lvclass">[])  [unwired: 1 in, 2 out]
              n73 = property class="Field"(reference=w196) -> ("goal_width"=w191:i32, "ourGoalPosition"=w195:dbl[])  [unwired: 1 in, 2 out]
              n74 = Equal?(x=-1) -> (x = y?=w193:bool)  [unwired: 1 in]
              n75 = feedback #3(-1 ("x")) -> (w186:i32)
              n76 = case shown="False" w193 {
                tunnel: w200 -> [w231 w276]
                tunnel: w180 -> [w230 w275]
                tunnel: w199 -> [w229 w274]
                tunnel: [w228 w273] -> w198
                tunnel: w197 -> [w227 w272]
                tunnel: w195 -> [w211 w256]
                tunnel: [w225 w270] -> w192
                tunnel: w191 -> [w220 w265]
                tunnel: w189 -> [w209 w254]
                tunnel: _ -> [w203 _]
                tunnel: [FALSE ("keepDest") FALSE ("keepDest")] -> w188
                tunnel: w186 -> [_ w248]
                tunnel: [w203 w248] -> w185
                frame False {
                  n77 = call "FindRobotByID.vi"("id"=w203, "RobotRef"=w229) -> ("Robot"=w226:refnum<class "Robot.lvclass">)  [unwired: 6 in, 3 out]
                  n78 = Divide(x=w220, y=2) -> (x/y=w213:dbl)
                  n79 = property class="Robot"(reference=w226) -> ("position(x,y)"=w224:dbl[])  [unwired: 1 in, 2 out]
                  n80 = Multiply(x=3.0, y=w209) -> (x*y=w205:dbl)
                  n81 = Divide(x=w205, y=w213) -> (x/y=w217:dbl)
                  n82 = Subtract(x=w224, y=w211) -> (x-y=w223:dbl[])
                  n83 = Inverse Cosine(1:w217) -> (0:w216:dbl)
                  n84 = Index Array(array=w223) -> (element #1=w222:dbl, element #2=w221:dbl)  [unwired: 2 in]
                  n85 = Inverse Tangent (2 Input)(1:w222, 2:w221) -> (0:w202:dbl)
                  n86 = Absolute Value(x=w202) -> (abs(x)=w215:dbl)
                  n87 = Negate(x=w202) -> (-x=w201:dbl)
                  n88 = Greater?(x=w215, y=w216) -> (0:w214:bool)
                  n89 = call-poly <vilib>:"2D Cartesian Coordinate Rotation.vi"("theta"=w201, "y"=0.0 ("element"), "x"=w213) -> ("y out"=w208:dbl, "x out"=w210:dbl)  [unwired: 6 in, 1 out]
                  n90 = case shown="False" w214 {
                    tunnel: w211 -> [w235 w243]
                    tunnel: w210 -> [_ w245]
                    tunnel: w208 -> [_ w244]
                    tunnel: [w232 w240] -> w207
                    tunnel: [w236 w239] -> w206
                    tunnel: w205 -> [w233 _]
                    tunnel: w202 -> [w238 _]
                    frame False {
                      n91 = Index Array(array=w235) -> (element=w234:dbl)  [unwired: 1 in]
                      n92 = Tangent(1:w238) -> (0:w237:dbl)
                      n93 = Add(x=w234, y=w233) -> (x+y=w232:dbl)
                      n94 = Multiply(x=w237, y=w233) -> (x*y=w236:dbl)
                    }
                    frame True {
                      n95 = Index Array(array=w243) -> (element #1=w242:dbl, element #2=w241:dbl)  [unwired: 2 in]
                      n96 = Add(x=w245, y=w242) -> (x+y=w240:dbl)
                      n97 = Add(x=w244, y=w241) -> (x+y=w239:dbl)
                    }
                  }
                  n98 = property class="Robot"(reference=w227, "dest_x"=w207, "dest_y"=w206, "dest_orientation"=w202) -> (reference out=w228:refnum<class "Robot.lvclass">)  [unwired: 1 in, 1 out]
                  n99 = call "DefendGoalTacticCheckStateChange.vi"("Game"=w230, "DefendGoalTactic in"=w231) -> ("States"=w225:T8)  [unwired: 7 in, 2 out]
                }
                frame True {
                  n100 = call "FindRobotByID.vi"("id"=w248, "RobotRef"=w274) -> ("Robot"=w271:refnum<class "Robot.lvclass">)  [unwired: 6 in, 3 out]
                  n101 = Divide(x=w265, y=2) -> (x/y=w258:dbl)
                  n102 = property class="Robot"(reference=w271) -> ("position(x,y)"=w269:dbl[])  [unwired: 1 in, 2 out]
                  n103 = Multiply(x=3.0, y=w254) -> (x*y=w250:dbl)
                  n104 = Divide(x=w250, y=w258) -> (x/y=w262:dbl)
                  n105 = Subtract(x=w269, y=w256) -> (x-y=w268:dbl[])
                  n106 = Inverse Cosine(1:w262) -> (0:w261:dbl)
                  n107 = Index Array(array=w268) -> (element #1=w267:dbl, element #2=w266:dbl)  [unwired: 2 in]
                  n108 = Inverse Tangent (2 Input)(1:w267, 2:w266) -> (0:w247:dbl)
                  n109 = Absolute Value(x=w247) -> (abs(x)=w260:dbl)
                  n110 = Negate(x=w247) -> (-x=w246:dbl)
                  n111 = Greater?(x=w260, y=w261) -> (0:w259:bool)
                  n112 = call-poly <vilib>:"2D Cartesian Coordinate Rotation.vi"("theta"=w246, "y"=0.0 ("element"), "x"=w258) -> ("y out"=w253:dbl, "x out"=w255:dbl)  [unwired: 6 in, 1 out]
                  n113 = case shown="True" w259 {
                    tunnel: w256 -> [w280 w288]
                    tunnel: w255 -> [_ w290]
                    tunnel: w253 -> [_ w289]
                    tunnel: [w277 w285] -> w252
                    tunnel: [w281 w284] -> w251
                    tunnel: w250 -> [w278 _]
                    tunnel: w247 -> [w283 _]
                    frame False {
                      n114 = Index Array(array=w280) -> (element=w279:dbl)  [unwired: 1 in]
                      n115 = Tangent(1:w283) -> (0:w282:dbl)
                      n116 = Add(x=w279, y=w278) -> (x+y=w277:dbl)
                      n117 = Multiply(x=w282, y=w278) -> (x*y=w281:dbl)
                    }
                    frame True {
                      n118 = Index Array(array=w288) -> (element #1=w287:dbl, element #2=w286:dbl)  [unwired: 2 in]
                      n119 = Add(x=w290, y=w287) -> (x+y=w285:dbl)
                      n120 = Add(x=w289, y=w286) -> (x+y=w284:dbl)
                    }
                  }
                  n121 = property class="Robot"(reference=w272, "dest_x"=w252, "dest_y"=w251, "dest_orientation"=w247) -> (reference out=w273:refnum<class "Robot.lvclass">)  [unwired: 1 in, 1 out]
                  n122 = call "DefendGoalTacticCheckStateChange.vi"("Game"=w275, "DefendGoalTactic in"=w276) -> ("States"=w270:T8)  [unwired: 7 in, 2 out]
                }
              }
              n123 = feedback-in #3(w185) -> ()
            }
            frame Enabled {
              n124 = property class="Game" props=["OffensiveTeam", "EnemyRef", "Parameters.lvclass", "Utilities.lvclass", "FieldRef", "BallRef"](reference=w293) -> ("OffensiveTeam"=w313:refnum<class "Ally.lvclass">, "EnemyRef"=w312:refnum<class "Enemy.lvclass">, "Parameters.lvclass"=w315:refnum<class "Parameters.lvclass">, "Utilities.lvclass"=w311:refnum<class "Utilities.lvclass">, "BallRef"=w299:refnum<class "Ball.lvclass">)  [unwired: 1 in, 3 out]
              n125 = property class="Parameters.lvclass"(reference=w315) -> ("AttakingOurselves"=w314:bool)  [unwired: 1 in, 2 out]
              n126 = call "FindReceiver.vi"("Game"=w293) -> ("Receiver Id"=w307:i32)  [unwired: 7 in, 3 out]
              n127 = Select(t=w313, s=w314, f=w312) -> (s? t:f=w310:refnum<class "Team.lvclass">)
              n128 = property class="Team"(reference=w310) -> ("RobotRef"=w309:refnum<class "Robot.lvclass">[])  [unwired: 1 in, 2 out]
              n129 = Not Equal?(x=w307, y=-1) -> (x != y?=w308:bool)
              n130 = feedback #4(-1 ("Receiver Id")) -> (w301:i32)
              n131 = Select(t=-1 ("Receiver Id"), s=w303, f=w301) -> (s? t:f=w300:i32)
              n132 = case shown="False" w308 {
                tunnel: w307 -> [w318 _]
                tunnel: w311 -> [w320 w329]
                tunnel: w309 -> [w319 w328]
                tunnel: [w318 w327] -> w305
                tunnel: w300 -> [_ w327]
                tunnel: [w316 w322] -> w291
                tunnel: w299 -> [_ w321]
                frame True {
                  n133 = call "FindRobotByID.vi"("id"=w318, "RobotRef"=w319, "Utilities in"=w320) -> ("Robot"=w317:refnum<class "Robot.lvclass">)  [unwired: 5 in, 3 out]
                  n134 = property class="Robot"(reference=w317) -> ("position(x,y)"=w316:dbl[])  [unwired: 1 in, 2 out]
                }
                frame False {
                  n135 = call "FindRobotByID.vi"("id"=w327, "RobotRef"=w328, "Utilities in"=w329) -> ("index"=w325:i32, "Robot"=w323:refnum<class "Robot.lvclass">)  [unwired: 5 in, 2 out]
                  n136 = Not Equal?(x=w325, y=-1) -> (x != y?=w326:bool)
                  n137 = case shown="False" w326 {
                    tunnel: w323 -> [_ w333]
                    tunnel: [w330 w332] -> w322
                    tunnel: w321 -> [w331 _]
                    frame False {
                      n138 = property class="Ball"(reference=w331) -> ("position(x,y)"=w330:dbl[])  [unwired: 1 in, 2 out]
                    }
                    frame True {
                      n139 = property class="Robot"(reference=w333) -> ("position(x,y)"=w332:dbl[])  [unwired: 1 in, 2 out]
                    }
                  }
                }
              }
              n140 = feedback-in #4(w305) -> ()
              n141 = call "BlockAngle.vi"("target"=w291, "Game ref"=w293, "Robot in"=w294, "DefendAreaTactic in"=w295) -> ("Robot out"=w292:refnum<class "Robot.lvclass">)  [unwired: 5 in, 2 out]
              n142 = call "DefendAreaTacticCheckStateChange.vi"("Game"=w293, "DefendAreaTactic in"=w297) -> ("States"=w296:T2)  [unwired: 7 in, 2 out]
            }
          }
        }
        frame "BlockPossibleShot" {
          n143 = property class="Game"(reference=w375) -> (reference out=w373:refnum<class "Game.lvclass">, "BallRef"=w374:refnum<class "Ball.lvclass">, "DefensiveTeam"=w372:refnum<class "Ally.lvclass">, "NewParameters"=w361:T5, "FieldRef"=w355:refnum<class "Field.lvclass">)  [unwired: 1 in, 1 out]
          n144 = property class="Skillbook"(reference=w357) -> ("HaltSkill"=w356:refnum<class "HaltSkill.lvclass">)  [unwired: 1 in, 2 out]
          n145 = property class="Field"(reference=w355) -> (reference out=w351:refnum<class "Field.lvclass">, "defense_stretch"=w354:i32, "defense_width_or_radius"=w336:i32, "field_length"=w338:i32)  [unwired: 1 in, 1 out]
          n146 = property class="Ball"(reference=w374) -> (reference out=w359:refnum<class "Ball.lvclass">, "position(x,y)"=w366:dbl[], "y"=w346:dbl, "x"=w340:dbl)  [unwired: 1 in, 1 out]
          n147 = property class="Ally"(reference=w372) -> ("RobotRef"=w367:refnum<class "Robot.lvclass">[])  [unwired: 1 in, 2 out]
          n148 = Divide(x=w338, y=2) -> (x/y=w335:dbl)
          n149 = Unbundle By Name(w361) -> ("RobotRadius"=w344:dbl, "Turning radius"=w360:dbl)  [unwired: 1 out]
          n150 = Divide(x=w354, y=2) -> (x/y=w345:dbl)
          n151 = property class="Robot"(reference=w371) -> ("id"=w370:i32, "position(x,y)"=w352:dbl[], "y"=w343:dbl)  [unwired: 1 in, 2 out]
          n152 = call "findRobotClosestToPosition.vi"("robotsArray"=w367, "position"=w366) -> ("id"=w365:i32)  [unwired: 5 in, 4 out]
          n153 = Subtract(x=w335, y=w336) -> (x-y=w334:dbl)
          n154 = call "BlockAngle.vi"("target"=w366, "Game ref"=w375, "Robot in"=w371, "DefendAreaTactic in"=w377) -> ("Robot out"=w376:refnum<class "Robot.lvclass">)  [unwired: 5 in, 2 out]
          n155 = Negate(x=w334) -> (-x=w339:dbl)
          n156 = Equal?(x=w365, y=w370) -> (x = y?=w358:bool)
          n157 = call "DefenseKick.vi"("object in"=w377, "Robot"=w376, "Game"=w375) -> ("Robot out"=w369:refnum<class "Robot.lvclass">)  [unwired: 14 in, 2 out]
          n158 = Multiply(x=3.0, y=w344) -> (x*y=w364:dbl)
          n159 = call "CheckWallState.vi"("Position"=w352, "Field"=w351) -> ("WallState"=w350:T4)  [unwired: 16 in, 1 out]
          n160 = Add(x=w364, y=w360) -> (x+y=w362:dbl)
          n161 = call "ElementAtGoalieArea.vi"("ElementRadius"=w362, "Elemento pos."=w366, "Game"=w373) -> ("Element at our goalkeeper area ?"=w347:bool)  [unwired: 4 in, 4 out]
          n162 = Equal?(x=w350, y=WallPositions."FrontWall") -> (x = y?=w348:bool)
          n163 = Add(x=w345, y=w344) -> (x+y=w342:dbl)
          n164 = case shown="True" w348 {
            tunnel: [w381 w395] -> w341
            tunnel: w347 -> [w383 w397]
            tunnel: w346 -> [w391 _]
            tunnel: w343 -> [w389 _]
            tunnel: w342 -> [w394 _]
            tunnel: w342 -> [w390 _]
            tunnel: w340 -> [_ w399]
            tunnel: w339 -> [_ w398]
            frame False {
              n165 = Greater Than 0?(x=w391) -> (x > 0?=w393:bool)
              n166 = Greater?(x=w389, y=w394) -> (0:w392:bool)
              n167 = Negate(x=w390) -> (-x=w388:dbl)
              n168 = Less Than 0?(x=w391) -> (x < 0?=w387:bool)
              n169 = And(x=w393, y=w392) -> (x .and. y?=w384:bool)
              n170 = Less?(x=w389, y=w388) -> (x < y?=w386:bool)
              n171 = And(x=w387, y=w386) -> (x .and. y?=w385:bool)
              n172 = Or(x=w384, y=w385) -> (x .or. y?=w382:bool)
              n173 = And(x=w383, y=w382) -> (x .and. y?=w381:bool)
            }
            frame True {
              n174 = Greater?(x=w399, y=w398) -> (0:w396:bool)
              n175 = And(x=w397, y=w396) -> (x .and. y?=w395:bool)
            }
          }
          n176 = case shown="True" w341 {
            tunnel: w369 -> [w400 w403]
            tunnel: [w400 w406] -> w368
            tunnel: w366 -> [_ w405]
            tunnel: w359 -> [_ w404]
            tunnel: w358 -> [_ w402]
            tunnel: w356 -> [_ w401]
            frame False {
            }
            frame True {
              n177 = case shown="True" w402 {
                tunnel: [w408 w416] -> w406
                tunnel: w405 -> [_ w415]
                tunnel: w404 -> [_ w411]
                tunnel: w403 -> [w407 w410]
                tunnel: w401 -> [w409 _]
                frame False {
                  n178 = call-dynamic "HaltSkill.vi"("Robot"=w407, "HaltSkill in"=w409) -> ("Robot out"=w408:refnum<class "Robot.lvclass">)  [unwired: 7 in, 2 out]
                }
                frame True {
                  n179 = Index Array(array=w415) -> (element #1=w414:dbl, element #2=w413:dbl)  [unwired: 2 in]
                  n180 = call "robotOrientatedToBall.vi"("Robot"=w410, "BallRef"=w411) -> ("Orientation"=w412:dbl)  [unwired: 7 in, 2 out]
                  n181 = property class="Robot"(reference=w410, "dest_orientation"=w412, "dest_x"=w414, "dest_y"=w413) -> (reference out=w416:refnum<class "Robot.lvclass">)  [unwired: 1 in, 1 out]
                }
              }
            }
          }
          n182 = call "DefendAreaTacticCheckStateChange.vi"("Game"=w375, "DefendAreaTactic in"=w377) -> ("States"=w379:T2)  [unwired: 7 in, 2 out]
        }
        frame "BallInKeeperArea" {
          n183 = property class="Skillbook"(reference=w420) -> ("HaltSkill"=w419:refnum<class "HaltSkill.lvclass">)  [unwired: 1 in, 2 out]
          n184 = call-dynamic "HaltSkill.vi"("Robot"=w418, "HaltSkill in"=w419) -> ("Robot out"=w417:refnum<class "Robot.lvclass">)  [unwired: 7 in, 2 out]
          n185 = call "DefendAreaTacticCheckStateChange.vi"("Game"=w421, "DefendAreaTactic in"=w422) -> ("States"=w423:T2)  [unwired: 7 in, 2 out]
        }
        frame "Exit" {
        }
      }
      n186 = feedback-in #2(w14) -> ()
      n187 = Or(x=w15, y=errorcluster {"status"=FALSE, "code"=0, "source"=""}) -> (x .or. y?=→"x .or. y?":bool)
      n188 = property class="DefendAreaTactic"(reference=w31, "States"=w14) -> (reference out=w21:refnum<class "DefendAreaTactic.lvclass">)  [unwired: 1 in, 1 out]
      n189 = property class="Robot"(reference=w27, "tactic"=tactics."DefendGoal", "keepDest"=w23, "robotKickState"=robotKickToStates."walk") -> (reference out=w20:refnum<class "Robot.lvclass">)  [unwired: 1 in, 1 out]
    }
    frame Error {
    }
  }
  "error out" <- w4
  "DefendAreaTactic out" <- w3
  "Robot out" <- w8
